vi "Eval LTFC (No Objects).vi"(8 "error in (no error)":errorcluster, 10 "Desired Field (T)":dbl) -> (0 "error out":errorcluster, 2 "Desired Control Voltage":dbl)   [LabVIEW 2009]
doc: "Evaluates Long-Term Field Calibration for control voltage that corresponds to desired field.\nAlso error checks to see if Long-Term Field Calibration is initialized properly."
uses:
  <vilib>/gmath/interp.llb/in_piecewise interp poly control.ctl
  <vilib>/Utility/error.llb/DialogType.ctl
  <vilib>/gmath/NI_Gmath.lvlib
panel:
  in  "piecewise polynomial":T1={"x locations"=[0.0, 0.027578469362999607, 0.026417725882999735, 0.02728830753199964, 0.026998129674999673, 0.026998129674999673, 0.02728830753199964, 0.02728830753199964, 0.02728830753199964, 0.02728830753199964, 0.02728830753199964, 0.026998129674999673, 0.02728830753199964, 0.026998129674999673, 0.027578469362999607, 0.026998129674999673, 0.027868615167999898, 0.026707935791999704, 0.027868615167999898, 0.02728830753199964, 0.028158744946999867, 0.026998129674999673, 0.028158744946999867, 0.027578469362999607, 0.028738956426999803, 0.028158744946999867, 0.02902903812799977, 0.02902903812799977, 0.029899187074999674, 0.029899187074999674, 0.031349114799999835, 0.03192897370799977, 0.033378340522999615, 0.03395797506699987, 0.03627587220299962, 0.037724037067999774, 0.04061916484799978, 0.04322340962699981, 0.046693716722999754, 0.04929493258799979, 0.05391611114799992, 0.057956276927999796, 0.0628579696669999, 0.06919446158699984, 0.07552319692299977, 0.08184417567499971, 0.08930442306699984, 0.09675383688299967, 0.10562167130799964, 0.11418878276799965, 0.12416551656299982, 0.13440681866699963, 0.14661226490799986, 0.15822241920299984, 0.1709342611679997, 0.18473913676299974, 0.19794439339199985, 0.21195367569199985, 0.22564390128299988, 0.24096464666799974, 0.2556824076269997, 0.2714607014879998, 0.2866360109229996, 0.3028610837879997, 0.3182095492279998, 0.3345985631479998, 0.35092988346799986, 0.3685570415229997, 0.3850378634719997, 0.40226511364799955, 0.41942672132799946, 0.43652268651199994, 0.4538185871469998, 0.4715758023679996, 0.4892610768749994, 0.5068744106679999, 0.5244158037469997, 0.5421454493229995, 0.5610962674999996, 0.578930173307, 0.5974581183469997, 0.6151361072, 0.6335013562879996, 0.651023428187, 0.6702347983229995, 0.6883496571869998, 0.7063814372669994, 0.7235839346999998, 0.7424433097719999, 0.7599783048029997, 0.7789038142519997, 0.796758438003, 0.8154988471519995, 0.8322114778429998, 0.8505312895469999, 0.8663655018749997, 0.8837977924479999, 0.8992478184029998, 0.9155745269879996, 0.9297096442679996, 0.9447235115319995, 0.9573404031999997, 0.9715366066669997, 0.9838225984119998, 0.9960635731229995, 1.006881116012, 1.0183502773119997], "coefficients"=[[9.0, -54.390255683024264, 1972.1999421765022, -23837.43535845014], [8.5, 0.0, -222663.3552147834, -127885479.75291832], [8.4, 0.0, -395824.10447629006, 303110841.608787], [8.3, 0.0, -3562810.4428854287, -8185348759.825917], [8.2, 0.0, nan, inf], [8.1, -1033.8486992135772, 7125620.885770729, -16370697519.651539], [8.0, -1033.8486992135772, nan, nan], [7.9, -inf, nan, nan], [7.8, -inf, nan, nan], [7.7, -inf, nan, nan], [7.6, 0.0, -3562810.4428853653, -8185348759.825771], [7.5, 0.0, -3562810.4428853653, 8185348759.825771], [7.4, 0.0, -3562810.442885397, -8185348759.825844], [7.3, 0.0, -890751.8046587084, 1023253361.2955427], [7.2, 0.0, -890751.8046587163, -1023253361.2955519], [7.1, 0.0, -395911.55674268235, 303211299.84458774], [7.0, 0.0, -222687.95116455198, -127906670.16183503], [6.9, 0.0, -222687.951164554, 127906670.16183618], [6.8, 0.0, -890850.2047597626, -1023422922.0210439], [6.7, 0.0, -395955.29374474613, 303261545.61010224], [6.6, 0.0, -222712.55119006446, -127927865.25273718], [6.5, 0.0, -222712.55119006446, 127927865.25273718], [6.4, 0.0, -890948.6211678976, -1023592520.2136359], [6.3, 0.0, -222761.76347155275, 127970269.48535071], [6.199999999999999, 0.0, -891145.502917806, -1023931829.038042], [6.1, 0.0, -5.820766091346741e-11, -151706174.76677823], [6.0, -344.7114220236917, nan, inf], [5.9, -344.768560640498, 792435.7360408008, -607126506.9219533], [5.8, -344.768560640498, nan, inf], [5.699999999999999, -206.90686496112463, 215092.062924836, -82733591.34830745], [5.6, -104.96108050107424, -349153.94803292025, 401400268.61249375], [5.5, -104.98504710205145, 74504.85168816571, -34272712.375057235], [5.4, -105.00170402698365, -395301.79652969027, 481015558.40565896], [5.3, -78.43351217720291, 35163.95141340095, -8601991.147578163], [5.199999999999999, -54.067056867428626, -35360.313850715094, 17271614.350897465], [5.1, -47.81705609199579, 9814.238960474726, -1805969.2413398365], [5.0, -36.401732973542764, -3549.680013267086, 1068567.2801981643], [4.9, -33.14884307521726, 3751.0220031768913, -721101.5684704564], [4.8, -33.167192891887005, -7905.262678054137, 2259266.174733769], [4.699999999999999, -28.433001621158166, 3261.78488959898, -387716.0974151777], [4.6, -23.125791409562083, -1377.8288914566833, 241438.6796169321], [4.5, -22.436138782793783, 318.79239369822835, 19661.584494672647], [4.3999999999999995, -17.893691470983697, 668.1684577129545, -52844.23096006572], [4.3, -15.791270141645406, -1.5262446928090976, -0.39506217726663984], [4.2, -15.81063600922985, -204.73102777028393, 32146.390232362693], [4.1, -14.545631848021925, 307.2610496986933, -20680.743695678033], [4.0, -13.414123393400958, -155.10733352518014, 20645.689962532426], [3.8999999999999995, -12.287919544471878, 250.1242096807369, -15346.821834752074], [3.8, -11.4723519561564, -147.87594640995093, 14533.28128408451], [3.6999999999999993, -10.806063460689025, 143.82341495431484, -6551.9013762498635], [3.5999999999999996, -9.892722391709318, -56.13841040363944, 6705.194646386277], [3.5, -8.932774920223483, 138.13213934111516, -6351.84779486039], [3.3999999999999995, -8.39960601942923, -69.90440901004814, 4436.766978397453], [3.3, -8.22863686622757, 31.77493996353212, -259.67858901323393], [3.1999999999999993, -7.546685946794582, 55.615464325476, -2439.4446336796723], [3.0999999999999996, -7.405845298541045, -42.05774137729267, 2227.8320186632413], [3.0, -7.351151795109956, 36.304112915912796, -1505.998160635863], [2.8999999999999995, -7.220664216504015, -41.70171438552485, 2598.882962828332], [2.8, -6.901210285879032, 57.4477892920075, -2155.8407625190225], [2.6999999999999993, -6.659015096198783, -34.28747745927314, 1704.1410293983552], [2.5999999999999996, -6.560870207430023, 36.14957018453386, -1395.1509862260757], [2.5, -6.462100712647977, -31.17102378520257, 1500.1917479063045], [2.3999999999999995, -6.371723028438886, 36.33825670520326, -1447.9165214990633], [2.3, -6.336046361163596, -37.129366901074214, 1658.1351683788507], [2.1999999999999993, -6.303956446873841, 25.345095908598374, -793.2733623870106], [2.0999999999999996, -6.112413332928348, -15.453666948722104, 905.8027332773754], [2.0, -5.892405463678817, 35.828650721685705, -1326.6620790090954], [1.8999999999999995, -5.8659390793181245, -32.57304699914481, 1233.761225660242], [1.7999999999999998, -5.934266865230393, 15.679067145382014, -473.7454112331958], [1.6999999999999993, -5.815844298949046, -0.6443906971513643, -0.1929713217308412], [1.5999999999999996, -5.83813236181487, -3.295594130476314, 154.44630175362002], [1.5, -5.815394086478147, -0.48601435999693043, 140.67710746752925], [1.3999999999999995, -5.705956297150455, 9.028657126866378, -272.3630667523945], [1.2999999999999998, -5.6429521798369615, -0.6450081410298454, -0.19943592573777996], [1.1999999999999993, -5.6659536039896015, -0.6529221385465761, -0.2035422770742736], [1.0999999999999996, -5.689143309596932, -3.0607311846165297, 136.59809144416496], [1.0, -5.670428395946461, -7.0755085506020485, 495.01754947640495], [0.8999999999999995, -5.454508970773896, 27.295804577857062, -945.5700318468864], [0.7999999999999998, -5.438710963940166, -24.870035905809146, 864.4734069258126], [0.6999999999999993, -5.500938095910305, 18.085635206759207, -674.0881609261595], [0.5999999999999996, -5.524971337818885, -20.97240419600133, 764.6738062889135], [0.5, -5.549563600375942, 18.40174714437124, -692.166111907913], [0.40000000000000036, -5.5740245488678255, -29.94753468542641, 1275.7342544951277], [0.29999999999999893, -5.448470972818899, 33.360127600797355, -1077.4821399084235], [0.1999999999999993, -5.359704249478379, -17.033202531678814, 450.79718470340964], [0.09999999999999964, -5.533027634495179, 5.884151192692265, -365.4930200015953], [0.0, -5.677338979744133, -31.083936956173403, 1348.1444983893043], [-0.09999999999999964, -5.549928976562321, 36.60949762442517, -1245.250920199711], [-0.20000000000000107, -5.497782186646598, -35.6448333583639, 1365.7408146817677], [-0.3000000000000007, -5.488048362199237, 29.786839160903064, -1003.8569128709298], [-0.40000000000000036, -5.439255222157796, -25.62752118272026, 928.6273284962755], [-0.5, -5.466290116734501, 30.51242818308866, -1257.3586983987848], [-0.5999999999999996, -5.647423536120942, -56.40323086089519, 2171.662477637961], [-0.7000000000000011, -5.713001940215277, 50.02625483131713, -1972.6175184990652], [-0.8000000000000007, -5.86618185217128, -75.61291815792441, 2983.4364287167905], [-0.9000000000000004, -6.016681902515738, 52.408191770170134, -2084.322116610954], [-1.0, -6.089673392705022, -61.00870941172982, 2345.0806748262007], [-1.1000000000000014, -6.295510178805808, 48.580706354740876, -2335.6197069877403], [-1.200000000000001, -6.576942377305138, -85.35265017996389, 3547.687219109779], [-1.3000000000000007, -6.863381703233459, 66.7216027095899, -3544.007387373401], [-1.4000000000000004, -7.256513272558122, -142.42358778415132, 7083.37502167763], [-1.5, -7.46767776859887, 96.38562097026725, -4687.930779080555], [-1.6000000000000014, -7.565364905308268, -92.22081072342135, 3703.5725747842034], [-1.700000000000001, -8.154299266522761, 39.65062935340357, -3339.1771027359077], [-1.8000000000000007, -8.684616099746068, -128.21579858572127, 7070.227007248946], [-1.9000000000000004, -8.976518251164514, 21.334314301080568, 97.29387558876765]]} {"x locations" format="%.4g"; "coefficients" format="%.4g"}
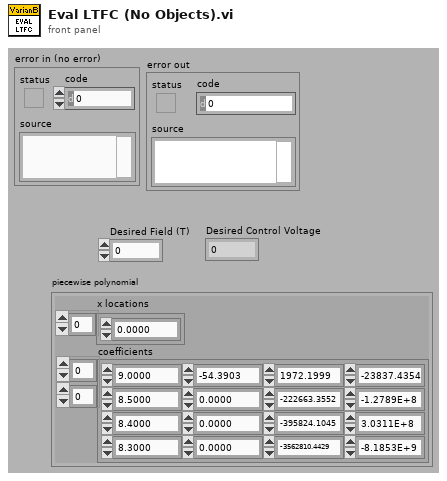
[diagram p1: front panel]
types:
  T1 = typedef "NI_Gmath.lvlib/in_piecewise interp poly control.ctl" = cluster{"x locations":dbl[], "coefficients":dbl[][]}
  T2 = typedef "DialogType.ctl" = u16
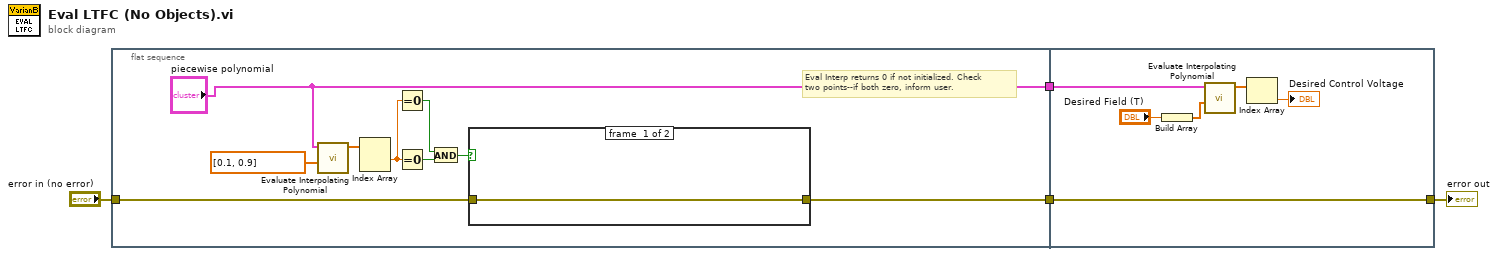
[diagram p0: block diagram]
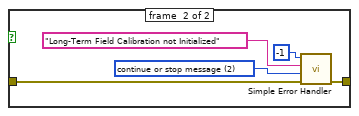
[diagram p2: hidden frame]
diagram:
  n1 = flat-sequence {
    tunnel: "error in (no error)" -> [w7]
    tunnel: [w6] -> w3
    tunnel: ["piecewise polynomial"] -> w2
    tunnel: [w25] -> w1
    tunnel: w3 -> [w25]
    tunnel: w2 -> [w23]
    frame #0 {
      # "Eval Interp returns 0 if not initialized. Check\ntwo points--if both zero, inform user."
      n2 = call <vilib>:"Evaluate Interpolating Polynomial.vi"("xi"=dbl[] [0.1, 0.9], "piecewise polynomial"="piecewise polynomial") -> ("yi"=w13:dbl[])  [unwired: 8 in, 1 out]
      n3 = Index Array(array=w13) -> (element #1=w11:dbl)  [unwired: 2 in, 1 out]
      n4 = Equal To 0?(x=w11) -> (x = 0?=w10:bool)
      n5 = Equal To 0?(x=w11) -> (x = 0?=w9:bool)
      n6 = And(x=w10, y=w9) -> (x .and. y?=w8:bool)
      n7 = case shown="True" w8 {
        tunnel: w7 -> [w14 w16]
        tunnel: [w14 w15] -> w6
        frame #0 {
        }
        frame #1 {
          w17 = T2 2 items=["no dialog", "OK message", "continue or stop message", "OK message + warnings", "continue/stop + warnings"] ("type of dialog (OK msg:1)")
          n8 = call <vilib>:"Simple Error Handler.vi"("error code (no error:0)"=-1, "error source (\" \")"="Long-Term Field Calibration not Initialized" ("error source (\" \")"), "type of dialog (OK msg:1)"=w17, "error in (no error)"=w16) -> ("error out"=w15:errorcluster)  [unwired: 1 in, 4 out]
        }
      }
    }
    frame #1 {
      n9 = Build Array("Desired Field (T)") -> (w21:dbl[])
      n10 = call <vilib>:"Evaluate Interpolating Polynomial.vi"("xi"=w21, "piecewise polynomial"=w23) -> ("yi"=w24:dbl[])  [unwired: 8 in, 1 out]
      n11 = Index Array(array=w24) -> (element=→"Desired Control Voltage":dbl)  [unwired: 1 in]
    }
  }
  "error out" <- w1
